vi "getDatabase.vi"(8 "error in (no error)":errorcluster, 11 "HWController in":refnum<class "HWController.lvclass">) -> (0 "error out":errorcluster, 2 "deviceDataBase":refnum<class "deviceDataBase.lvclass">, 3 "HWController out":refnum<class "HWController.lvclass">)   [LabVIEW 2009, in "Hardware.lvlib" / "HWControllers.lvlib" / "HWController.lvclass"]
uses:
  HWController.lvclass
  Tools/DatabaseHelpers/DbConnection/DeviceDataBase/deviceDataBase.lvclass
  HWController.lvclass/HWController.ctl
  Tools/DatabaseHelpers.lvlib
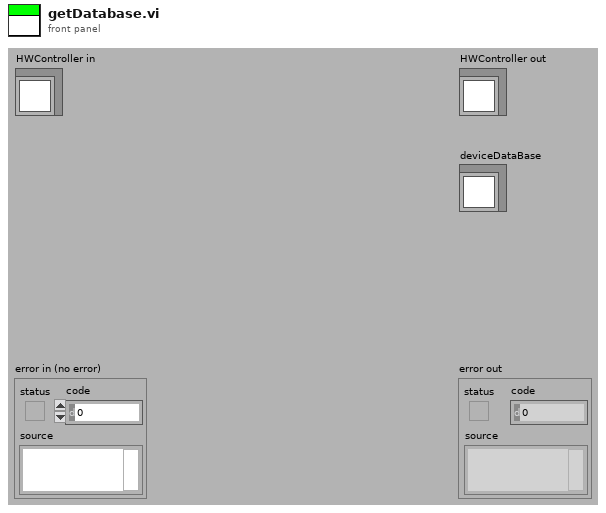
[diagram p1: front panel]
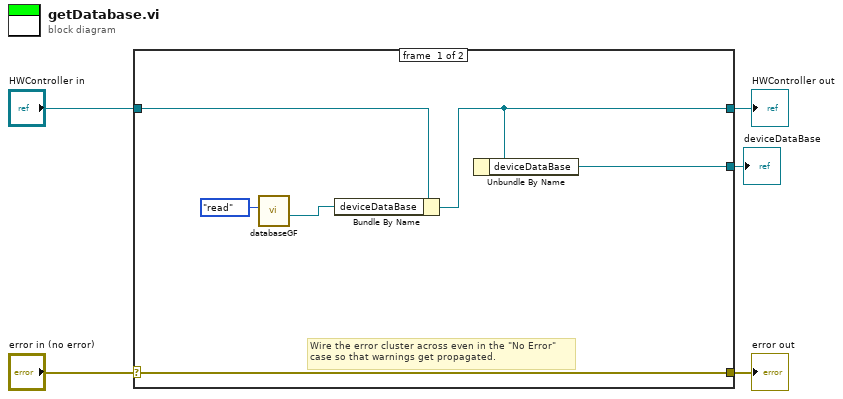
[diagram p0: block diagram]
diagram:
  n1 = case shown="No Error" "error in (no error)" {
    selector: "error in (no error)" -> [w11 w13]
    tunnel: [w11 w13] -> w4
    tunnel: [w6 w12] -> w2
    tunnel: "HWController in" -> [w7 w12]
    tunnel: [w10 _] -> w1
    frame #0 {
      # "Wire the error cluster across even in the \"No Error\"\ncase so that warnings get propagated."
      n2 = call "databaseGF.vi"("Enum"=enum16{"write", "read"}."read") -> ("deviceDataBase out"=w8:refnum<class "deviceDataBase.lvclass">)  [unwired: 10 in]
      n3 = Bundle By Name(cluster=w7, "deviceDataBase"=w8) -> (w6:refnum<class "HWController.lvclass">)
      n4 = Unbundle By Name(w6) -> ("deviceDataBase"=w10:refnum<class "deviceDataBase.lvclass">)
    }
    frame #1 {
    }
  }
  "error out" <- w4
  "HWController out" <- w2
  "deviceDataBase" <- w1
